vi "Event_ball_possession.vi"(8 "error in (no error)":errorcluster, 10 "Game":refnum<class "Game.lvclass">, 11 "Events in":refnum<class "Events.lvclass">) -> (0 "error out":errorcluster, 3 "Events out":refnum<class "Events.lvclass">)   [LabVIEW 2023, in "Events.lvclass"]
uses:
  Events.lvclass
  Game_class/Game.lvclass
  Game_class/Game.lvclass/Game.ctl
  Parameters_class/Parameters.lvclass/Parameters.ctl
  Team_class/Team.lvclass/Team.ctl
  Possession.ctl
  Events.lvclass/Events.ctl
  Write id_our_balll_possesion.vi
  Write id_enemy_ball_possesion.vi
  Game_class/Read Parameters.lvclass.vi
  Game_class/Read BallRef.vi
  Game_class/Read AllyRef.vi
  Game_class/Read EnemyRef.vi
  Team_class/Read RobotRef.vi
  Parameters_class/Read DistanceForPossession.vi
  Enemy_class/Enemy.lvclass
  C:/Users/ebert/Desktop/roboime/SSL_AI/Team_class/Team.lvclass
  Ally_class/Ally.lvclass
  Parameters_class/Parameters.lvclass
  Ball_class/Ball.lvclass
  Robot_class/Robot.lvclass
panel:
  in  "TimeThreshold":dbl=0.1
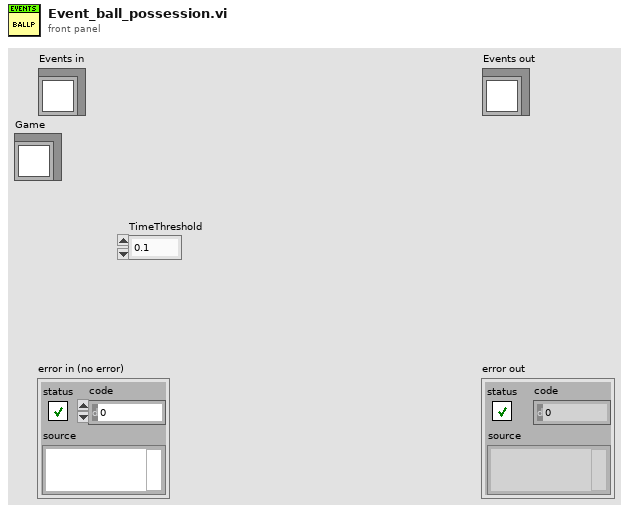
[diagram p1: front panel]
types:
  T1 = typedef "Events.lvclass/Possession.ctl" = enum16{"OurPossession", "TheirPossession", "Contended", "Loose"}
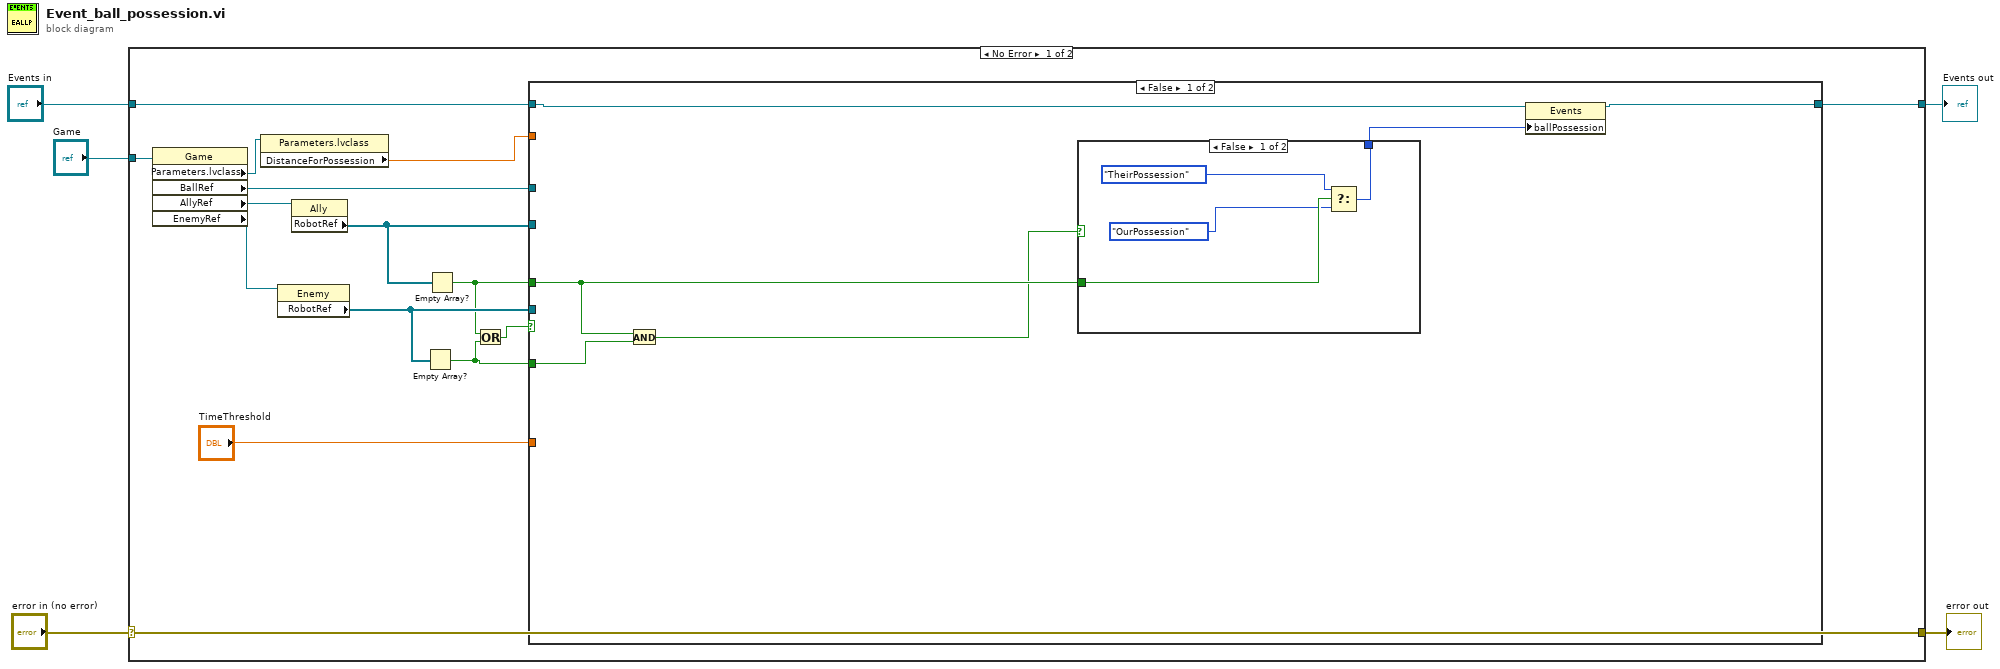
[diagram p0: block diagram]
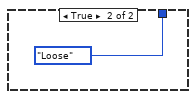
[diagram p2: hidden frame]
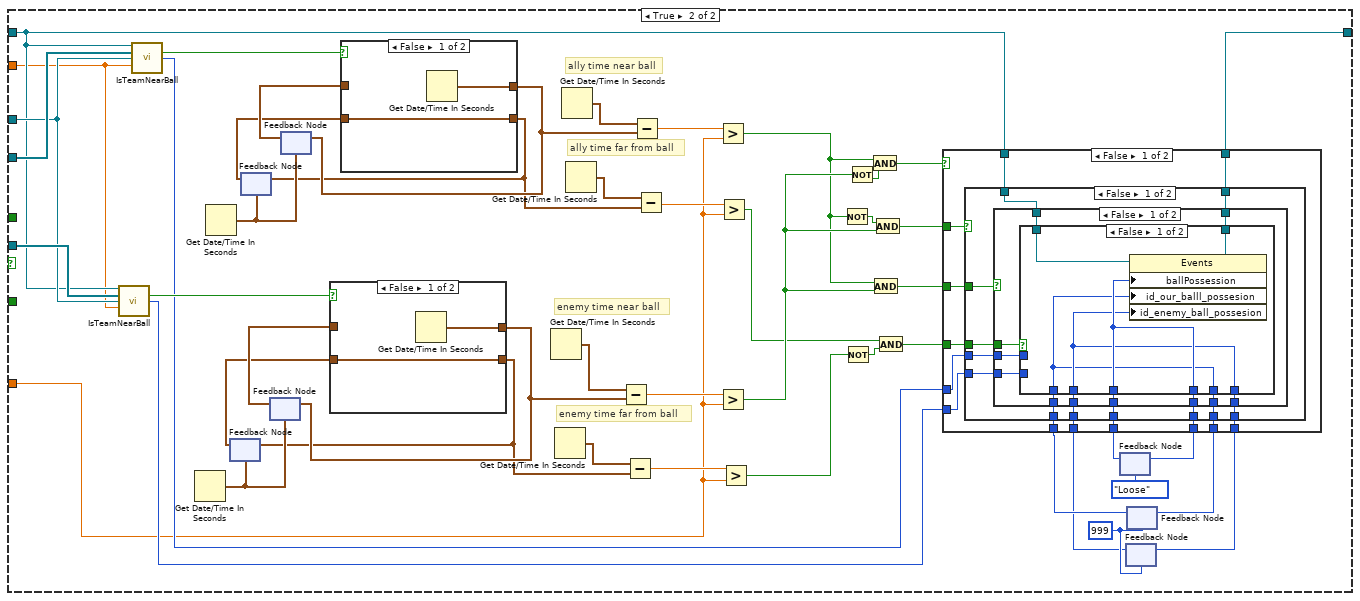
[diagram p3: hidden frame]
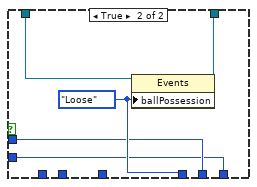
[diagram p4: hidden frame]
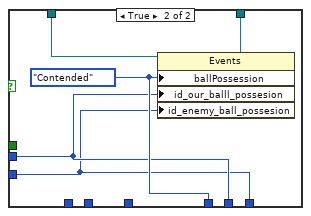
[diagram p5: hidden frame]
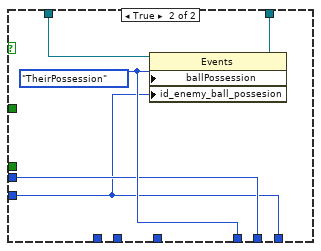
[diagram p6: hidden frame]
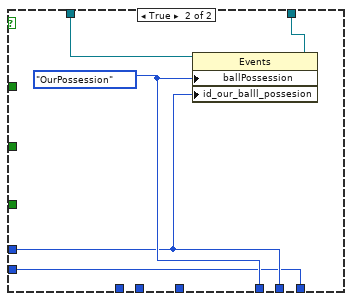
[diagram p7: hidden frame]
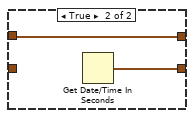
[diagram p8: hidden frame]
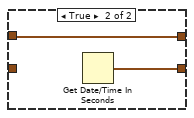
[diagram p9: hidden frame]
diagram:
  n1 = case shown="No Error" "error in (no error)" {
    selector: "error in (no error)" -> [w20 w150]
    tunnel: [w20 w150] -> w4
    tunnel: [w14 w149] -> w2
    tunnel: "Events in" -> [w15 w149]
    tunnel: "Game" -> [w19 _]
    frame No Error {
      n2 = property class="Game"(reference=w19) -> ("Parameters.lvclass"=w13:refnum<class "Parameters.lvclass">, "BallRef"=w16:refnum<class "Ball.lvclass">, "AllyRef"=w17:refnum<class "Ally.lvclass">, "EnemyRef"=w18:refnum<class "Enemy.lvclass">)  [unwired: 1 in, 2 out]
      n3 = property class="Parameters.lvclass"(reference=w13) -> ("DistanceForPossession"=w12:dbl)  [unwired: 1 in, 2 out]
      n4 = property class="Enemy"(reference=w18) -> ("RobotRef"=w10:refnum<class "Robot.lvclass">[])  [unwired: 1 in, 2 out]
      n5 = property class="Ally"(reference=w17) -> ("RobotRef"=w9:refnum<class "Robot.lvclass">[])  [unwired: 1 in, 2 out]
      n6 = Empty Array?(array=w10) -> (empty?=w6:bool)
      n7 = Empty Array?(array=w9) -> (empty?=w7:bool)
      n8 = Or(x=w7, y=w6) -> (x .or. y?=w8:bool)
      n9 = case shown="False" w8 {
        tunnel: w10 -> [_ w79]
        tunnel: w9 -> [_ w78]
        tunnel: w16 -> [_ w60]
        tunnel: w15 -> [w26 w48]
        tunnel: [w25 w34] -> w14
        tunnel: w12 -> [_ w33]
        tunnel: "TimeThreshold" -> [_ w32]
        tunnel: w7 -> [w23 _]
        tunnel: w6 -> [w22 _]
        frame False {
          n10 = And(x=w23, y=w22) -> (x .and. y?=w21:bool)
          n11 = case shown="False" w21 {
            tunnel: w23 -> [w30 _]
            tunnel: [w27 Possession."Loose" ("ballPossession")] -> w24
            frame False {
              n12 = Select(t=Possession."TheirPossession" ("ballPossession"), s=w30, f=Possession."OurPossession" ("ballPossession")) -> (s? t:f=w27:T1)
            }
            frame True {
            }
          }
          n13 = property class="Events"(reference=w26, "ballPossession"=w24) -> (reference out=w25:refnum<class "Events.lvclass">)  [unwired: 1 in, 1 out]
        }
        frame True {
          w38 = 999
          # "enemy time far from ball"
          # "enemy time near ball"
          # "ally time far from ball"
          # "ally time near ball"
          n14 = call-dynamic "IsTeamNearBall.vi"("Events in"=w48, "TeamRobots"=w79, "Ball"=w60, "DistanceToBallPos"=w33) -> ("possession"=w61:bool, "idPossession"=w41:i32)  [unwired: 8 in, 2 out]
          n15 = call-dynamic "IsTeamNearBall.vi"("Events in"=w48, "TeamRobots"=w78, "Ball"=w60, "DistanceToBallPos"=w33) -> ("possession"=w73:bool, "idPossession"=w40:i32)  [unwired: 8 in, 2 out]
          n16 = Get Date/Time In Seconds() -> (seconds since 1Jan1904=w65:timestamp)
          n17 = Get Date/Time In Seconds() -> (seconds since 1Jan1904=w72:timestamp)
          n18 = feedback #1(w65) -> (w64:timestamp)
          n19 = feedback #2(w72) -> (w71:timestamp)
          n20 = feedback #3(w65) -> (w68:timestamp)
          n21 = feedback #4(w72) -> (w77:timestamp)
          n22 = case shown="False" w61 {
            tunnel: w68 -> [_ w144]
            tunnel: [w142 w144] -> w66
            tunnel: w64 -> [w141 _]
            tunnel: [w141 w143] -> w62
            frame False {
              n23 = Get Date/Time In Seconds() -> (seconds since 1Jan1904=w142:timestamp)
            }
            frame True {
              n24 = Get Date/Time In Seconds() -> (seconds since 1Jan1904=w143:timestamp)
            }
          }
          n25 = feedback-in #1(w62) -> ()
          n26 = feedback-in #3(w66) -> ()
          n27 = case shown="False" w73 {
            tunnel: w77 -> [_ w148]
            tunnel: [w146 w148] -> w75
            tunnel: w71 -> [w145 _]
            tunnel: [w145 w147] -> w69
            frame False {
              n28 = Get Date/Time In Seconds() -> (seconds since 1Jan1904=w146:timestamp)
            }
            frame True {
              n29 = Get Date/Time In Seconds() -> (seconds since 1Jan1904=w147:timestamp)
            }
          }
          n30 = feedback-in #2(w69) -> ()
          n31 = feedback-in #4(w75) -> ()
          n32 = Get Date/Time In Seconds() -> (seconds since 1Jan1904=w67:timestamp)
          n33 = Get Date/Time In Seconds() -> (seconds since 1Jan1904=w63:timestamp)
          n34 = Get Date/Time In Seconds() -> (seconds since 1Jan1904=w76:timestamp)
          n35 = Get Date/Time In Seconds() -> (seconds since 1Jan1904=w70:timestamp)
          n36 = Subtract(x=w67, y=w66) -> (x-y=w58:dbl)
          n37 = Subtract(x=w63, y=w62) -> (x-y=w57:dbl)
          n38 = Subtract(x=w76, y=w75) -> (x-y=w74:dbl)
          n39 = Subtract(x=w70, y=w69) -> (x-y=w59:dbl)
          n40 = Greater?(x=w74, y=w32) -> (0:w52:bool)
          n41 = Greater?(x=w58, y=w32) -> (0:w53:bool)
          n42 = Greater?(x=w59, y=w32) -> (0:w51:bool)
          n43 = Greater?(x=w57, y=w32) -> (0:w49:bool)
          n44 = Not(x=w52) -> (.not. x?=w54:bool)
          n45 = Not(x=w49) -> (.not. x?=w50:bool)
          n46 = Not(x=w53) -> (.not. x?=w56:bool)
          n47 = And(x=w52, y=w56) -> (x .and. y?=w55:bool)
          n48 = And(x=w52, y=w53) -> (x .and. y?=w46:bool)
          n49 = And(x=w54, y=w53) -> (x .and. y?=w47:bool)
          n50 = And(x=w51, y=w50) -> (x .and. y?=w45:bool)
          n51 = feedback #5(Possession."Loose" ("ballPossession")) -> (w42:T1)
          n52 = feedback #6(w38) -> (w35:i32)
          n53 = feedback #7(w38) -> (w39:i32)
          n54 = case shown="False" w55 {
            tunnel: w48 -> [w90 w140]
            tunnel: [w91 w139] -> w34
            tunnel: w47 -> [w92 _]
            tunnel: w46 -> [w89 _]
            tunnel: w45 -> [w88 _]
            tunnel: [w87 w138] -> w43
            tunnel: w42 -> [w86 _]
            tunnel: w41 -> [w85 w136]
            tunnel: w40 -> [w84 w137]
            tunnel: w39 -> [w83 _]
            tunnel: w35 -> [w82 _]
            tunnel: [w81 w137] -> w37
            tunnel: [w80 w136] -> w36
            frame False {
              n55 = case shown="False" w92 {
                tunnel: [w102 w135] -> w91
                tunnel: w90 -> [w103 w134]
                tunnel: w89 -> [w104 _]
                tunnel: w88 -> [w101 _]
                tunnel: [w100 w133] -> w87
                tunnel: w86 -> [w99 _]
                tunnel: w85 -> [w97 w131]
                tunnel: w84 -> [w98 w132]
                tunnel: w83 -> [w96 _]
                tunnel: w82 -> [w95 _]
                tunnel: [w94 w132] -> w81
                tunnel: [w93 w131] -> w80
                frame False {
                  n56 = case shown="False" w104 {
                    tunnel: w103 -> [w114 w130]
                    tunnel: [w113 w129] -> w102
                    tunnel: w101 -> [w115 _]
                    tunnel: [w112 w128] -> w100
                    tunnel: w99 -> [w111 _]
                    tunnel: w98 -> [w108 w127]
                    tunnel: w97 -> [w107 w126]
                    tunnel: w96 -> [w110 _]
                    tunnel: w95 -> [w109 _]
                    tunnel: [w106 w127] -> w94
                    tunnel: [w105 w126] -> w93
                    frame False {
                      n57 = case shown="False" w115 {
                        tunnel: w114 -> [w120 w125]
                        tunnel: [w119 w124] -> w113
                        tunnel: [w118 w123] -> w112
                        tunnel: w111 -> [w118 _]
                        tunnel: w110 -> [w116 _]
                        tunnel: w109 -> [w117 _]
                        tunnel: w108 -> [_ w122]
                        tunnel: w107 -> [_ w121]
                        tunnel: [w116 w122] -> w106
                        tunnel: [w117 w121] -> w105
                        frame False {
                          n58 = property class="Events"(reference=w120, "ballPossession"=w118, "id_our_balll_possesion"=w116, "id_enemy_ball_possesion"=w117) -> (reference out=w119:refnum<class "Events.lvclass">)  [unwired: 1 in, 1 out]
                        }
                        frame True {
                          w123 = Possession."Loose" ("ballPossession")
                          n59 = property class="Events"(reference=w125, "ballPossession"=w123) -> (reference out=w124:refnum<class "Events.lvclass">)  [unwired: 1 in, 1 out]
                        }
                      }
                    }
                    frame True {
                      w128 = Possession."Contended" ("ballPossession")
                      n60 = property class="Events"(reference=w130, "ballPossession"=w128, "id_our_balll_possesion"=w127, "id_enemy_ball_possesion"=w126) -> (reference out=w129:refnum<class "Events.lvclass">)  [unwired: 1 in, 1 out]
                    }
                  }
                }
                frame True {
                  w133 = Possession."TheirPossession" ("ballPossession")
                  n61 = property class="Events"(reference=w134, "ballPossession"=w133, "id_enemy_ball_possesion"=w131) -> (reference out=w135:refnum<class "Events.lvclass">)  [unwired: 1 in, 1 out]
                }
              }
            }
            frame True {
              w138 = Possession."OurPossession" ("ballPossession")
              n62 = property class="Events"(reference=w140, "ballPossession"=w138, "id_our_balll_possesion"=w137) -> (reference out=w139:refnum<class "Events.lvclass">)  [unwired: 1 in, 1 out]
            }
          }
          n63 = feedback-in #5(w43) -> ()
          n64 = feedback-in #6(w36) -> ()
          n65 = feedback-in #7(w37) -> ()
        }
      }
    }
    frame Error {
    }
  }
  "error out" <- w4
  "Events out" <- w2
